vi "FTW-Endpoint-TCP-Send-Worker.vi"(0 "TCP Endpoint":refnum<class "FTW-Endpoint-TCP.lvclass">, 5 "Address":string) -> ()   [LabVIEW 2013, in "FTW-Endpoint-TCP.lvclass"]
uses:
  FTW-Endpoint-TCP.lvclass
  FTW-Endpoint-TCP.lvclass/FTW-Endpoint-TCP.ctl
panel:
  out "connected":bool
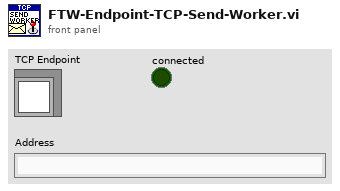
[diagram p1: front panel]
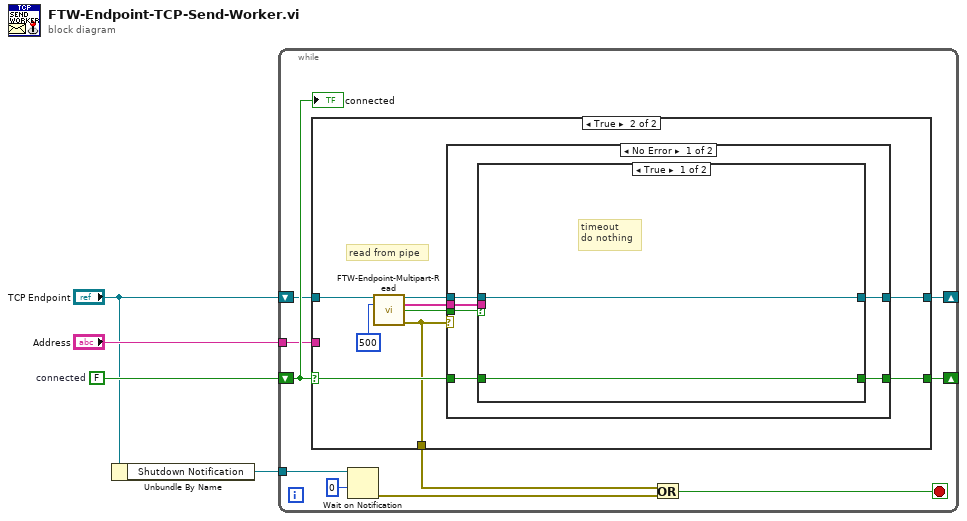
[diagram p0: block diagram]
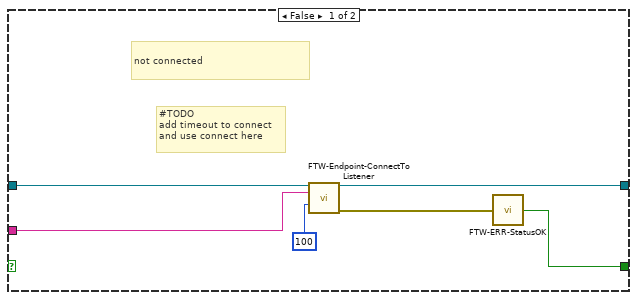
[diagram p2: hidden frame]
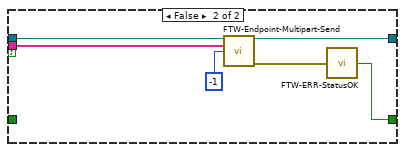
[diagram p3: hidden frame]
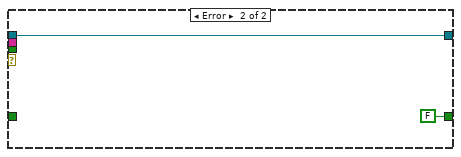
[diagram p4: hidden frame]
diagram:
  w4 = FALSE  # connected
  n1 = Unbundle By Name("TCP Endpoint") -> ("Shutdown Notification"=w1:refnum<notifier>)
  n2 = while {
    shift-right: [w11] -> _
    shift-left: w4 -> [w14]
    shift-right: [w12] -> _
    shift-left: "TCP Endpoint" -> [w7]
    tunnel: "Address" -> [w13]
    tunnel: w1 -> [w9]
    stop <- w6 stop-if-true
    n3 = case shown="True" w14 {
      selector: w14 -> [_ w26]
      tunnel: w13 -> [w20 _]
      tunnel: [w15 w28] -> w12
      tunnel: [w19 w27] -> w11
      tunnel: w7 -> [w16 w29]
      tunnel: [_ w24] -> w5
      frame False {
        # "not connected"
        # "#TODO\nadd timeout to connect\nand use connect here"
        n4 = call-dynamic "FTW-Endpoint-ConnectToListener.vi"("FTW-Endpoint In"=w16, "Address"=w20, "Timeout"=100) -> ("FTW-Endpoint Out"=w15:refnum<class "FTW-Endpoint-TCP.lvclass">, "error out"=w18:errorcluster)  [unwired: 10 in, 1 out]
        n5 = call "FTW-ERR-StatusOK.vi"("error to check"=w18) -> ("Status OK?"=w19:bool)
      }
      frame True {
        # "read from pipe"
        n6 = call-dynamic "FTW-Endpoint-Multipart-Read.vi"("FTW Endpoint"=w29, "Timeout"=500) -> ("FTW Endpoint out"=w25:refnum<class "FTW-Endpoint-TCP.lvclass">, "Message Received"=w21:string[], "Timed out?"=w22:bool, "error out"=w24:errorcluster)  [unwired: 10 in]
        n7 = case shown="No Error" w24 {
          tunnel: [w35 w45] -> w28
          tunnel: [w34 FALSE ("Status OK?")] -> w27
          tunnel: w26 -> [w33 _]
          tunnel: w25 -> [w32 w45]
          tunnel: w22 -> [w31 _]
          tunnel: w21 -> [w30 _]
          frame No Error {
            n8 = case shown="True" w31 {
              tunnel: w32 -> [w37 w43]
              tunnel: [w37 w42] -> w35
              tunnel: [w36 w40] -> w34
              tunnel: w33 -> [w36 _]
              tunnel: w30 -> [_ w38]
              frame True {
                # "timeout\ndo nothing"
              }
              frame False {
                n9 = call-dynamic "FTW-Endpoint-Multipart-Send.vi"("FTW Endpoint"=w43, "Multipart Message"=w38, "Timeout"=-1) -> ("FTW Endpoint out"=w42:refnum<class "FTW-Endpoint-TCP.lvclass">, "error out"=w41:errorcluster)  [unwired: 10 in, 1 out]
                n10 = call "FTW-ERR-StatusOK.vi"("error to check"=w41) -> ("Status OK?"=w40:bool)
              }
            }
          }
          frame Error {
          }
        }
      }
    }
    n11 = Wait on Notification(notifier=w9, timeout in ms (-1)=0) -> (error out=w8:errorcluster)  [unwired: 2 in, 3 out]
    n12 = Or(x=w5, y=w8) -> (x .or. y?=w6:bool)
    "connected" <- w14
  }
